vi "testimureset.vi"() -> ()   [LabVIEW 2017]
panel:
  out "yaw":dbl(graph)
  in  "Rset":bool
  in  "stop":bool
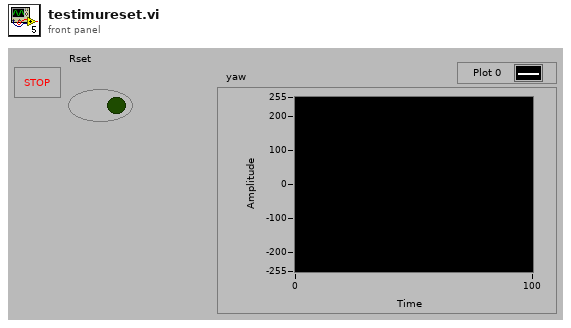
[diagram p1: front panel]
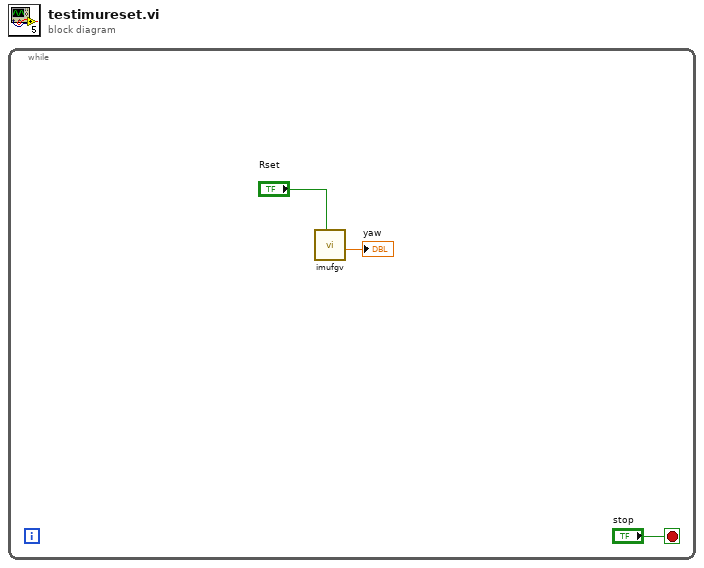
[diagram p0: block diagram]
diagram:
  n1 = while {
    stop <- "stop" stop-if-true
    n2 = call "imufgv.vi"("Rset"="Rset") -> ("yaw"=→"yaw":dbl)  [unwired: 9 in, 1 out]
  }
